vi "ДШ Семисег.vi"(1 "Cluster":T2) -> (0 "Cluster 2":T1)   [LabVIEW 2017]
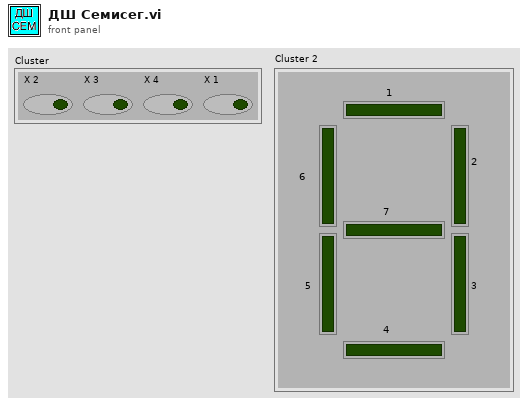
[diagram p1: front panel]
types:
  T1 = cluster{"1":bool, "2\n ":bool, "3 ":bool, "4":bool, "5 ":bool, "6":bool, "7":bool}
  T2 = cluster{"X 2":bool, "X 3":bool, "X 4":bool, "X 1":bool}
  T3 = cluster{bool, bool, bool, bool, bool, bool, bool}
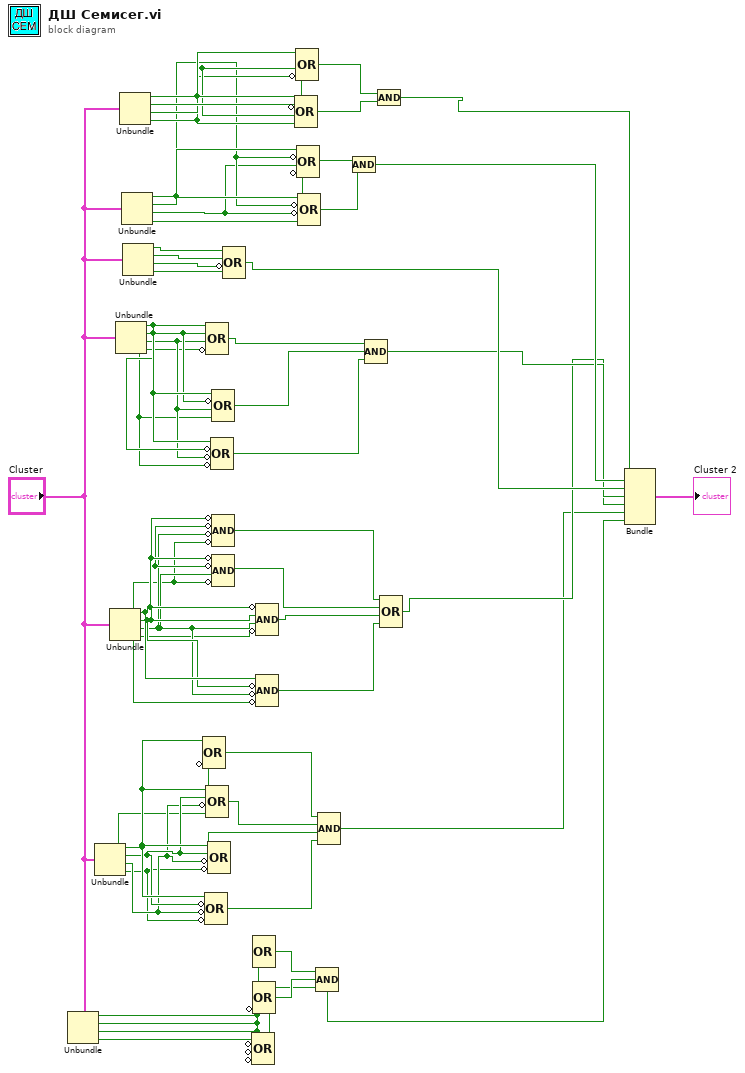
[diagram p0: block diagram]
diagram:
  n1 = Unbundle("Cluster") -> ("X 2"=w21:bool, "X 3"=w20:bool, "X 4"=w19:bool, "X 1"=w18:bool)
  n2 = Unbundle("Cluster") -> ("X 2"=w29:bool, "X 3"=w28:bool, "X 4"=w27:bool, "X 1"=w26:bool)
  n3 = Unbundle("Cluster") -> ("X 2"=w37:bool, "X 3"=w36:bool, "X 4"=w35:bool, "X 1"=w34:bool)
  n4 = Unbundle("Cluster") -> ("X 2"=w13:bool, "X 3"=w12:bool, "X 4"=w11:bool, "X 1"=w10:bool)
  n5 = Unbundle("Cluster") -> ("X 2"=w55:bool, "X 3"=w54:bool, "X 4"=w53:bool, "X 1"=w52:bool)
  n6 = Unbundle("Cluster") -> ("X 2"=w49:bool, "X 3"=w48:bool, "X 4"=w47:bool, "X 1"=w46:bool)
  n7 = Unbundle("Cluster") -> ("X 2"=w43:bool, "X 3"=w42:bool, "X 4"=w41:bool, "X 1"=w40:bool)
  n8 = Compound Arithmetic op=OR(w29, w28, w27, invert w26) -> (w25:bool)
  n9 = Compound Arithmetic op=OR(w29, invert w28, invert w27, invert w26) -> (w22:bool)
  n10 = Compound Arithmetic op=OR(w13, w12, w11, invert w10) -> (w39:bool)
  n11 = Compound Arithmetic op=OR(w29, w28, invert w27, w26) -> (w24:bool)
  n12 = Compound Arithmetic op=OR(w29, w28, invert w27, invert w26) -> (w23:bool)
  n13 = Compound Arithmetic op=OR(w13, invert w12, invert w11, invert w10) -> (w9:bool)
  n14 = Compound Arithmetic op=OR(w13, invert w12, w11, w10) -> (w38:bool)
  n15 = Compound Arithmetic op=AND(invert w37, invert w36, invert w35, invert w34) -> (w33:bool)
  n16 = Compound Arithmetic op=AND(invert w37, invert w36, w35, invert w34) -> (w32:bool)
  n17 = Compound Arithmetic op=OR(w43, w42, invert w41, w40) -> (w7:bool)
  n18 = Compound Arithmetic op=OR(w21, invert w20, invert w19, invert w18) -> (w15:bool)
  n19 = Compound Arithmetic op=OR(w21, w20, w19, w18) -> (w17:bool)
  n20 = Compound Arithmetic op=OR(w21, w20, w19, invert w18) -> (w16:bool)
  n21 = Compound Arithmetic op=AND(invert w37, w36, w35, invert w34) -> (w31:bool)
  n22 = Compound Arithmetic op=AND(w37, invert w36, invert w35, invert w34) -> (w30:bool)
  n23 = Compound Arithmetic op=OR(w55, invert w54, w53, w52) -> (w50:bool)
  n24 = Compound Arithmetic op=OR(w55, w54, w53, invert w52) -> (w51:bool)
  n25 = Compound Arithmetic op=OR(w49, invert w48, w47, invert w46) -> (w45:bool)
  n26 = Compound Arithmetic op=OR(w49, invert w48, invert w47, w46) -> (w44:bool)
  n27 = Compound Arithmetic op=AND(w17, w16, w15) -> (w1:bool)
  n28 = Compound Arithmetic op=AND(w25, w24, w23, w22) -> (w4:bool)
  n29 = Compound Arithmetic op=AND(w45, w44) -> (w8:bool)
  n30 = Compound Arithmetic op=AND(w39, w38, w9) -> (w6:bool)
  n31 = Compound Arithmetic op=AND(w51, w50) -> (w2:bool)
  n32 = Compound Arithmetic op=OR(w33, w32, w31, w30) -> (w5:bool)
  n33 = Bundle(w2, w8, w7, w6, w5, w4, w1) -> (→"Cluster 2":T3)  [unwired: 1 in]
